vi "Detect Tags.vi"(8 "error in (no error)":errorcluster, 10 "Greyscale Image":T4, 11 "Apriltag Detector in":refnum<class "AprilTag Detector.lvclass">) -> (0 "error out":errorcluster, 1 "# Detections":i32, 2 "Detections":T1[](array[typedef]), 3 "Apriltag Detector (Duplicate)":refnum<class "AprilTag Detector.lvclass">)   [LabVIEW 2020, in "g_ar_toolkit.feature_detection.lvlib" / "AprilTag Detector.lvclass"]
uses:
  AprilTag Detector.lvclass
  g_ar_toolkit.image/Greyscale Image.ctl
  Detection.ctl
  g_ar_toolkit.common/Image Point (Float).ctl
  g_ar_toolkit.common/Square Corners.ctl
  AprilTag Detector.lvclass/AprilTag Detector.ctl
  g_ar_toolkit.common/g_ar_toolkit.common.lvlib
  g_ar_toolkit.image/g_ar_toolkit.image.lvlib
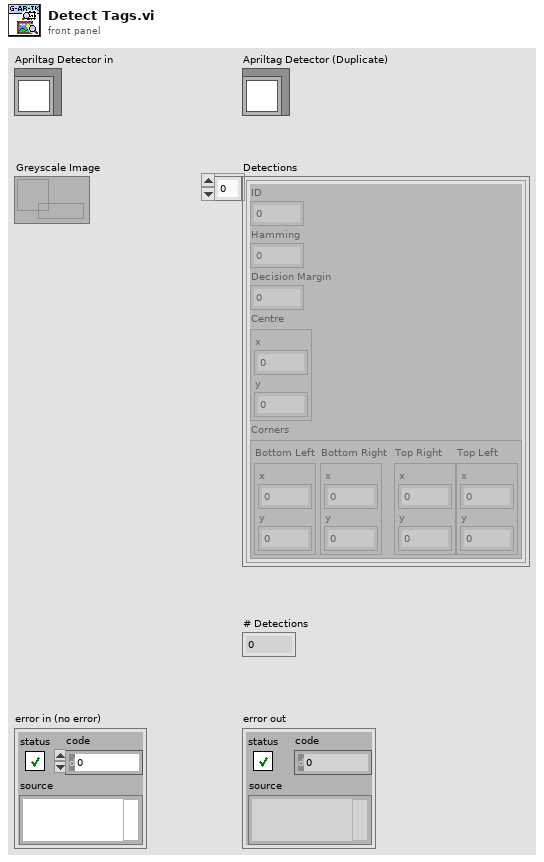
[diagram p1: front panel]
types:
  T1 = typedef "g_ar_toolkit.feature_detection.lvlib/AprilTag Detector.lvclass/Detection.ctl" = cluster{"ID":i32, "Hamming":i32, "Decision Margin":sgl, "Centre":T2, "Corners":T3}
  T2 = typedef "g_ar_toolkit.common.lvlib/Image Point (Float).ctl" = cluster{"x":dbl, "y":dbl}
  T3 = typedef "g_ar_toolkit.common.lvlib/Square Corners.ctl" = cluster{"Bottom Left":T2, "Bottom Right":T2, "Top Right":T2, "Top Left":T2}
  T4 = typedef "g_ar_toolkit.image.lvlib/Greyscale Image.ctl" = refnum<data-value>
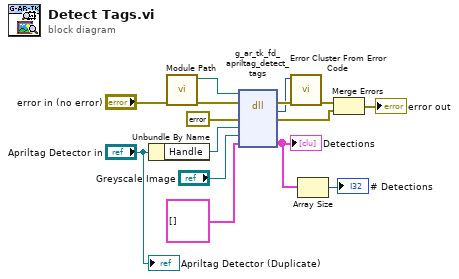
[diagram p0: block diagram]
diagram:
  n1 = Unbundle By Name("Apriltag Detector in") -> ("Handle"=w8:refnum<data-value>)
  n2 = call "Module Path.vi"("error in (no error)"="error in (no error)") -> ("error out"=w4:errorcluster, "Path"=w3:path)  [unwired: 9 in]
  n3 = dll-call lib="?" fn="g_ar_tk_fd_apriltag_detect_tags" ("g_ar_toolkit.*.*:g_ar_tk_capture_context_create")(path in=w3, error in=w4, "error_cluster"=errorcluster {"status"=FALSE, "code"=0, "source"=""} ("error constant"), "Detector_EDVR"=w8, "Image_EDVR"="Greyscale Image", "Detections"=T1[] [] ("Array")) -> (error out=w13:errorcluster, "MgErr"=w12:i32, "error_cluster"=w9:errorcluster, "Detections"=w2:T1[])  [unwired: 3 in, 1 out]
  "Detections" <- w2
  n4 = call <vilib>:"Error Cluster From Error Code.vi"("error in (no error)"=w13, "error code (0)"=w12) -> ("error out"=w11:errorcluster)  [unwired: 7 in]
  n5 = Array Size(array=w2) -> (size(s)=→"# Detections":i32)
  n6 = Merge Errors(w11, w9) -> (→"error out":errorcluster)
  "Apriltag Detector (Duplicate)" <- "Apriltag Detector in"
